vi "Signal.vi"(8 "error in (no error)":errorcluster, 11 "Signaller in":refnum<class "Signaller.lvclass">) -> (0 "error out":errorcluster, 3 "Signaller out":refnum<class "Signaller.lvclass">)   [LabVIEW 2015, in "Signaller.lvclass"]
uses:
  Signaller.lvclass
  Signaller.lvclass/Signaller.ctl
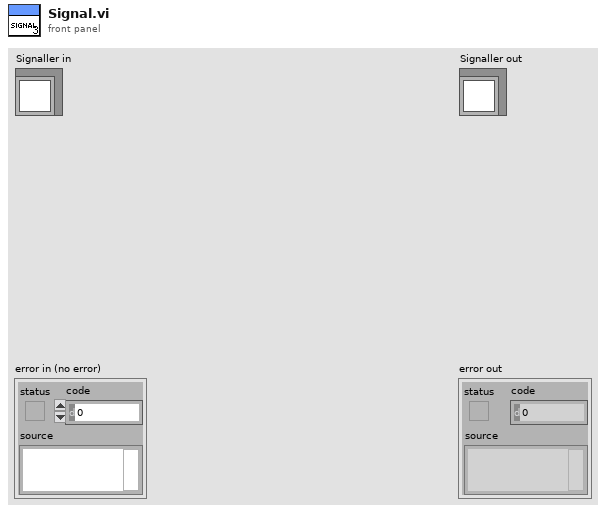
[diagram p1: front panel]
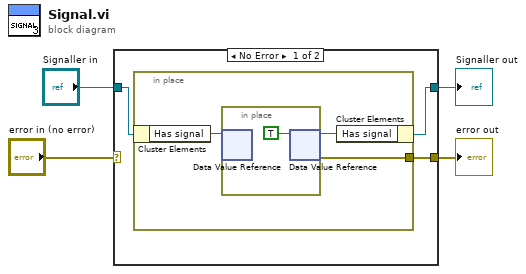
[diagram p0: block diagram]
diagram:
  n1 = case shown="No Error" "error in (no error)" {
    selector: "error in (no error)" -> [_ w13]
    tunnel: [w5 w13] -> w3
    tunnel: [w6 w12] -> w1
    tunnel: "Signaller in" -> [w7 w12]
    frame No Error {
      n2 = in-place {
        in-place-border: [w8] -> w5
        n3 = in-place-cluster #1(w7) -> ("Has signal"=w10:refnum<data-value>)
        n4 = in-place {
          n5 = in-place-dvr #2(w10) -> ()  [unwired: 2 out]
          n6 = in-place-dvr #2(TRUE ("data value")) -> (w9:refnum<data-value>, w8:errorcluster)
        }
        n7 = in-place-cluster #1("Has signal"=w9) -> (w6:refnum<class "Signaller.lvclass">)
      }
    }
    frame Error {
    }
  }
  "error out" <- w3
  "Signaller out" <- w1
